vi "NCC Setup Results Array - IMAQ.vi"(0 "Image Ref 01":T1, 2 "Half Shift":i32, 11 "Image Ref 02":T1) -> (4 "NCC Results Array":dbl[](array[numeric]), 8 "Result Rows":i32, 15 "Result Columns":i32)   [LabVIEW 2016]
uses:
  <vilib>/vision/Image Controls.llb/IMAQ Image.ctl
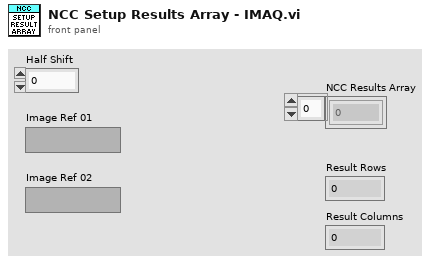
[diagram p1: front panel]
types:
  T1 = typedef "IMAQ Image.ctl" = refnum<image>
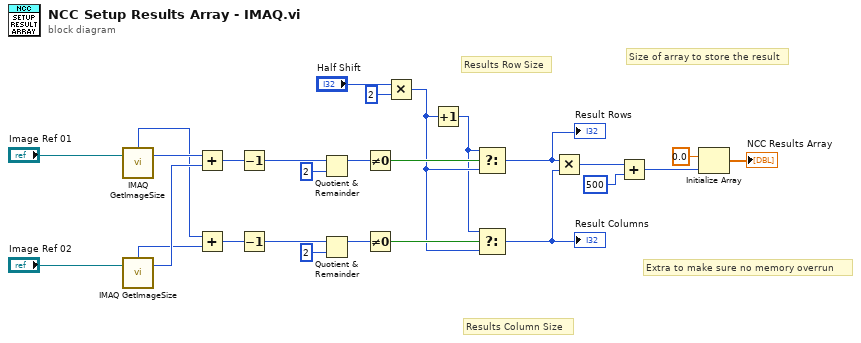
[diagram p0: block diagram]
diagram:
  # "Extra to make sure no memory overrun"
  # "Size of array to store the result"
  # "Results Column Size"
  # "Results Row Size"
  n1 = call "IMAQ GetImageSize"("Image"="Image Ref 01") -> ("Y Resolution"=w25:i32, "X Resolution"=w15:i32)  [unwired: 3 in, 1 out]
  n2 = call "IMAQ GetImageSize"("Image"="Image Ref 02") -> ("Y Resolution"=w24:i32, "X Resolution"=w16:i32)  [unwired: 3 in, 1 out]
  n3 = Add(x=w25, y=w24) -> (x+y=w23:i32)
  n4 = Add(x=w15, y=w16) -> (x+y=w14:i32)
  n5 = Decrement(x=w23) -> (x-1=w22:i32)
  n6 = Decrement(x=w14) -> (x-1=w13:i32)
  n7 = Quotient & Remainder(x=w22, y=2) -> (x-y*floor(x/y)=w20:i32)  [unwired: 1 out]
  n8 = Quotient & Remainder(x=w13, y=2) -> (x-y*floor(x/y)=w11:i32)  [unwired: 1 out]
  n9 = Not Equal To 0?(x=w20) -> (x != 0?=w19:bool)
  n10 = Not Equal To 0?(x=w11) -> (x != 0?=w10:bool)
  n11 = Multiply(x="Half Shift", y=2) -> (x*y=w9:i32)
  n12 = Increment(x=w9) -> (x+1=w8:i32)
  n13 = Select(t=w8, s=w19, f=w9) -> (s? t:f=w7:i32)
  "Result Rows" <- w7
  n14 = Select(t=w8, s=w10, f=w9) -> (s? t:f=w6:i32)
  "Result Columns" <- w6
  n15 = Multiply(x=w7, y=w6) -> (x*y=w5:i32)
  n16 = Add(x=w5, y=500) -> (x+y=w3:i32)
  n17 = Initialize Array(0.0 ("element"), w3) -> (→"NCC Results Array":dbl[])
